vi "setDAQmx.AO_Config.vi"(8 "error in (no error)":errorcluster, 10 "DAQmx.AO.Config":T1={"output terminal configuration"=-1} {"output terminal configuration" items=["Default"=-1, "RSE"=10083, "Differential"=10106, "Pseudodifferential"=12529]}, 11 "DAQmx.AO in":refnum<class "DAQmx.AO.lvclass">) -> (0 "error out":errorcluster, 3 "DAQmx.AO out":refnum<class "DAQmx.AO.lvclass">)   [LabVIEW 2020, in "DAQmx.AO.lvclass"]
uses:
  DAQmx.AO.lvclass
  Typedefs/DAQmx.AO_Config.ctl
  Typedefs/AO.Terminal-enum.ctl
  DAQmx.AO.lvclass/DAQmx.AO.ctl
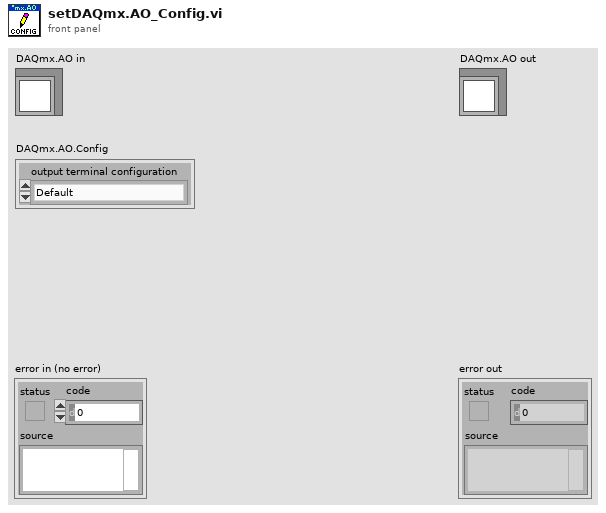
[diagram p1: front panel]
types:
  T1 = typedef "DAQmx.AO.lvclass/DAQmx.AO_Config.ctl" = cluster{"output terminal configuration":T2}
  T2 = typedef "DAQmx.AO.lvclass/AO.Terminal-enum.ctl" = i32
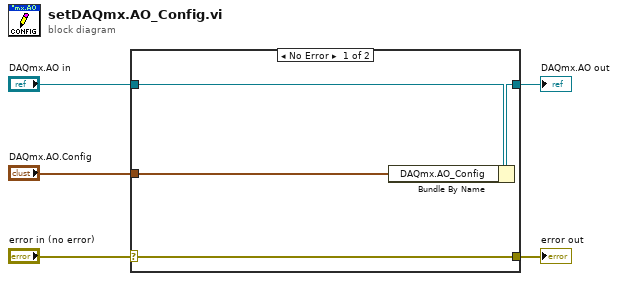
[diagram p0: block diagram]
diagram:
  n1 = case shown="No Error" "error in (no error)" {
    selector: "error in (no error)" -> [w9 w10]
    tunnel: [w9 w10] -> w4
    tunnel: [w7 w11] -> w2
    tunnel: "DAQmx.AO in" -> [w8 w11]
    tunnel: "DAQmx.AO.Config" -> [w6 _]
    frame No Error {
      n2 = Bundle By Name(cluster=w8, "DAQmx.AO_Config"=w6) -> (w7:refnum<class "DAQmx.AO.lvclass">)
    }
    frame Error {
    }
  }
  "error out" <- w4
  "DAQmx.AO out" <- w2
